vi "Build Padding String.vi"(11 "Nesting Level":i32) -> (3 "Padding":string)   [LabVIEW 2026, in "VILab.lvlib"]
uses:
  VILab.lvlib
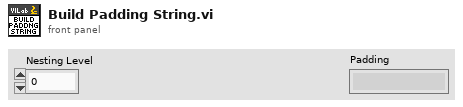
[diagram p1: front panel]
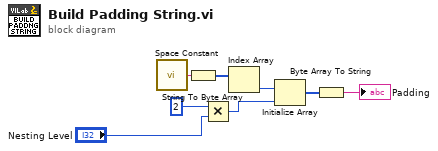
[diagram p0: block diagram]
diagram:
  n1 = call <vilib>:"Space Constant.vi"() -> ("String"=w7:string)
  n2 = String To Byte Array(string=w7) -> (unsigned byte array=w6:u8[])
  n3 = Multiply(x=2 ("y"), y="Nesting Level") -> (x*y=w3:i32)
  n4 = Index Array(array=w6) -> (element=w5:u8)  [unwired: 1 in]
  n5 = Initialize Array(w5, w3) -> (w4:u8[])
  n6 = Byte Array To String(unsigned byte array=w4) -> (string=→"Padding":string)
